vi "Filter Method Types.vi"(7 "VI Type to filter for":T2, 8 "Error in":errorcluster caption="Error in (no error)", 9 "Scope":T9, 11 "Methods":T1[](array[typedef])) -> (0 "Error out":errorcluster, 1 "All Filtered?":bool, 3 "Filtered Methods":T1[](array[typedef]))   [LabVIEW 2023, in "VIDoc Printer - Confluence.lvlib" / "VIDoc Printer - Confluence.lvclass"]
uses:
  VIDoc Printer - Confluence.lvclass
  Parsing/TypeDefs/VI Type Extended Enum.ctl
  Settings/Printer Settings/Scope Settings.ctl
  Parsing/TypeDefs/Method Spec Cluster.ctl
  <vilib>/picture/picture.llb/imagedata.ctl
  Parsing/TypeDefs/Class Dispatch Type Enum.ctl
  Parsing/TypeDefs/Controls Info Cluster.ctl
  <vilib>/Utility/miscctls.llb/LVKeyTypeDef.ctl
  <vilib>/Utility/miscctls.llb/LVPointTypeDef.ctl
  Parsing/SubVIs/Structure Reporter/Tree Cluster.ctl
  VIDoc Printer - Confluence.lvclass/VIDoc Printer - Confluence.ctl
  Parsing/VIDoc Parsing.lvlib
  Settings/Printer Settings/Printer Settings.lvclass
  Parsing/SubVIs/Structure Reporter/Structure Reporter.lvlib
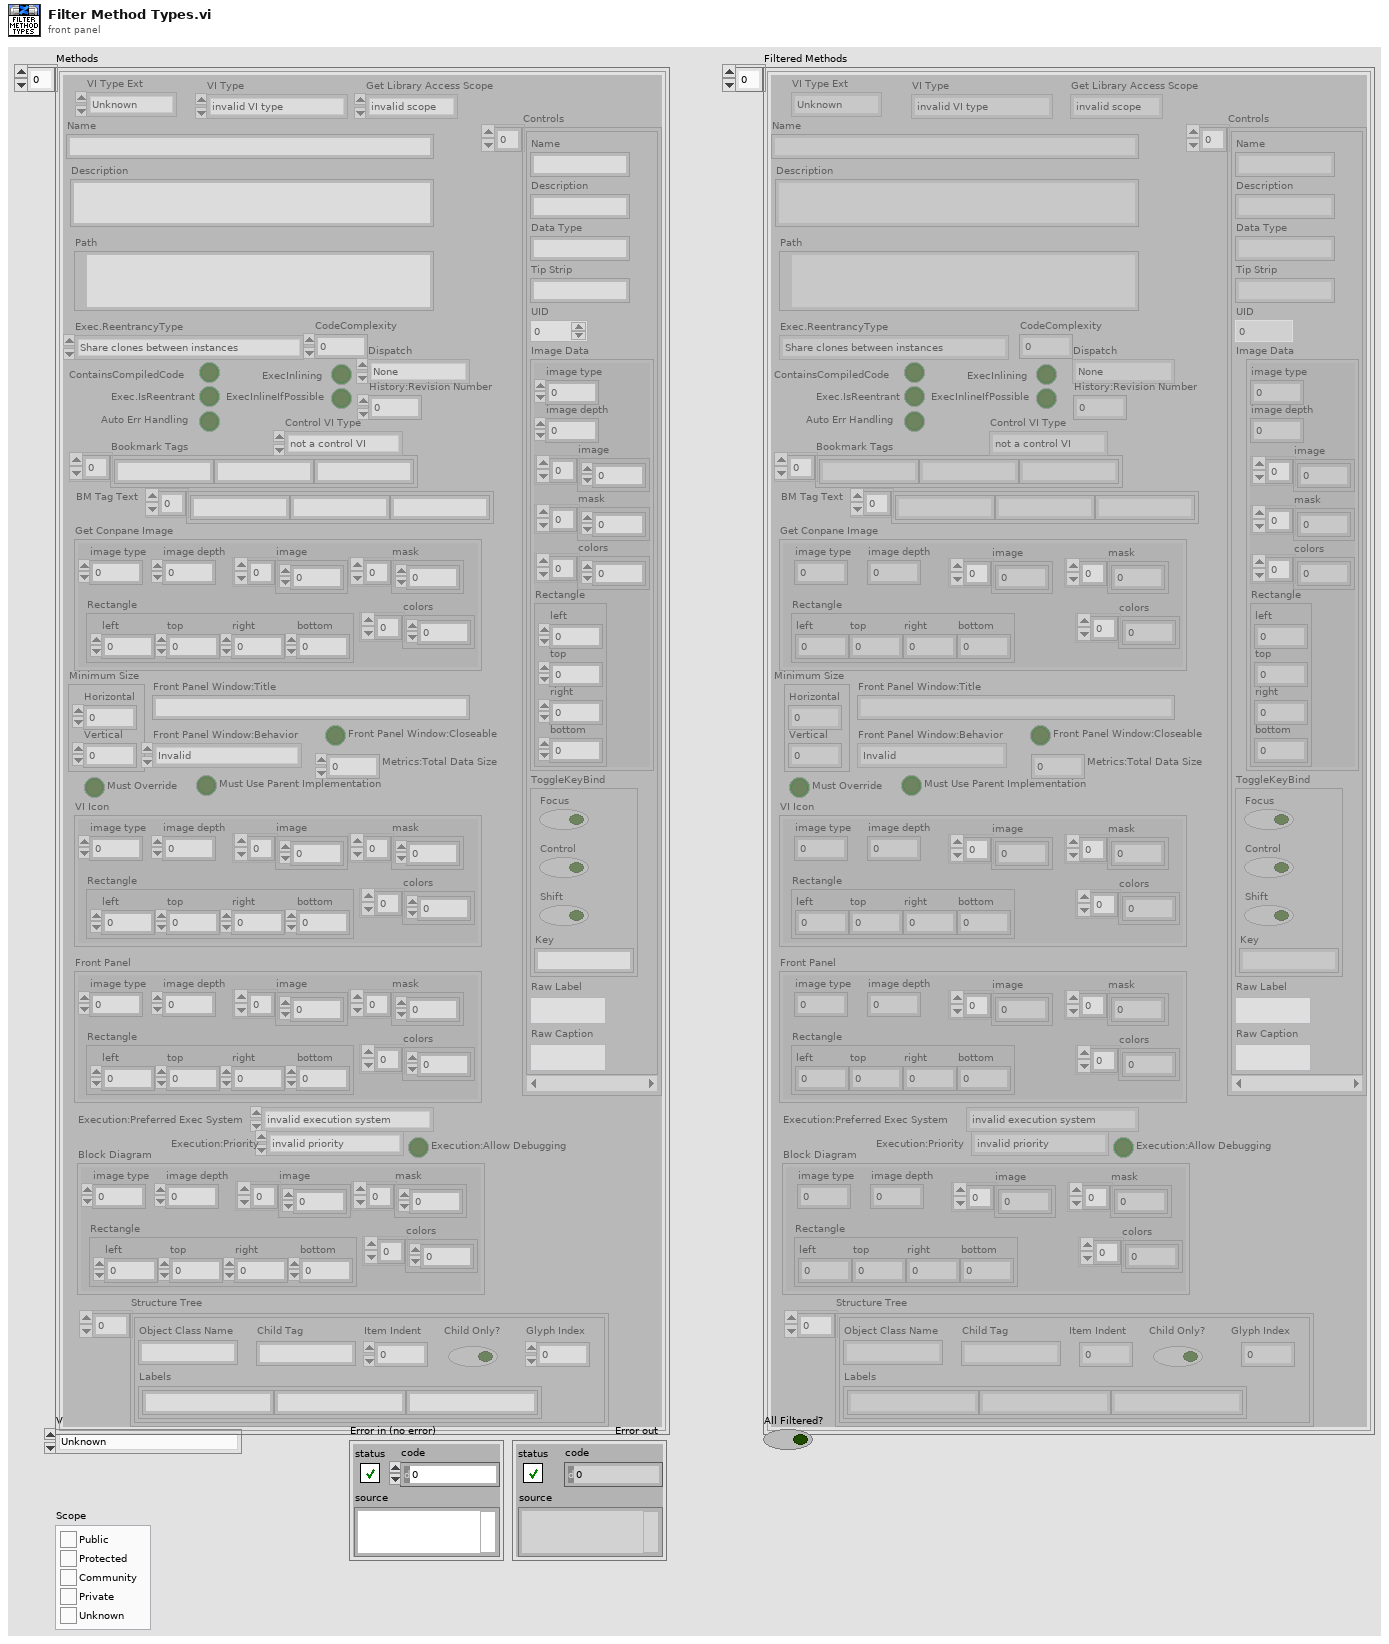
[diagram p1: front panel]
types:
  T1 = typedef "VIDoc Parsing.lvlib/Method Spec Cluster.ctl" = cluster{"VI Type Ext":T2, "Name":string, "Path":path, "Get Conpane Image":T3, "Description":string, "Get Library Access Scope":enum32{"invalid scope", "public", "private", "protected", "community"}, "Dispatch":T4, "ContainsCompiledCode":bool, "Exec.IsReentrant":bool, "Exec.ReentrancyType":enum16{"Share clones between instances", "Preallocate clone for each instance"}, "ExecInlining":bool, "ExecInlineIfPossible":bool, "Auto Err Handling":bool, "CodeComplexity":sgl, "Bookmark Tags":string[], "Control VI Type":enum32{"not a control VI", "control", "typedef", "strict typedef"}, "Controls":T5[], "VI Type":enum32{"invalid VI type", "Standard VI", "Control VI", "Global VI", "Polymorphic VI", "Configuration VI", "SubSystem", "Facade VI", "Method VI", "Statechart Diagram VI"}, "Minimum Size":T7, "Front Panel Window:Title":string, "Front Panel Window:Behavior":enum32{"Invalid", "Default", "Floating", "Floating/Auto-Hide", "Modal"}, "Front Panel Window:Closeable":bool, "Must Override":bool, "Must Use Parent Implementation":bool, "VI Icon":T3, "Front Panel":T3, "History:Revision Number":u32, "Metrics:Total Data Size":u32, "Execution:Allow Debugging":bool, "Execution:Preferred Exec System":enum32{"invalid execution system", "user interface", "standard", "instrument i/o", "data acquisition", "other 1", "other 2", "same as caller"}, "Execution:Priority":enum32{"invalid priority", "background priority", "normal priority", "above normal priority", "high priority", "time critical priority", "subroutine"}, "BM Tag Text":string[], "Block Diagram":T3, "Structure Tree":T8[]}
  T2 = typedef "VIDoc Parsing.lvlib/VI Type Extended Enum.ctl" = enum16{"Unknown", "Class Method", "Class Accessor Get", "Class Accessor Set", "Class Control", "Library Method", "Library Control", "VI", "Control"}
  T3 = typedef "imagedata.ctl" = cluster{"image type":i32, "image depth":i32, "image":u8[], "mask":u8[], "colors":u32[], "Rectangle":cluster{"left":i16, "top":i16, "right":i16, "bottom":i16}}
  T4 = typedef "VIDoc Parsing.lvlib/Class Dispatch Type Enum.ctl" = enum16{"None", "Static", "Dynamic"}
  T5 = typedef "VIDoc Parsing.lvlib/Controls Info Cluster.ctl" = cluster{"Name":string, "Description":string, "Data Type":string, "Tip Strip":string, "UID":i32, "Image Data":T3, "ToggleKeyBind":T6, "Raw Label":string, "Raw Caption":string}
  T6 = typedef "LVKeyTypeDef.ctl" = cluster{"Focus":bool, "Control":bool, "Shift":bool, "Key":string}
  T7 = typedef "LVPointTypeDef.ctl" = cluster{"Horizontal":i16, "Vertical":i16}
  T8 = typedef "VIDoc Parsing.lvlib/Structure Reporter.lvlib/Tree Cluster.ctl" = cluster{"Object Class Name":string, "Labels":string[], "Child Tag":string, "Item Indent":i32, "Child Only?":bool, "Glyph Index":i32}
  T9 = typedef "VIDoc Printer.lvlib/Printer Settings.lvclass/Scope Settings.ctl" = cluster{"Public":bool, "Protected":bool, "Community":bool, "Private":bool, "Unknown":bool}
  T10 = enum32{"invalid scope", "public", "private", "protected", "community"}
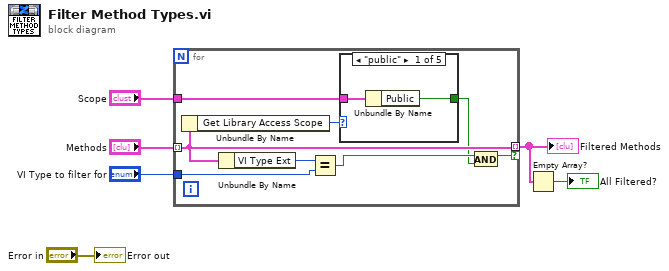
[diagram p0: block diagram]
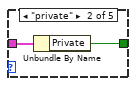
[diagram p2: hidden frame]
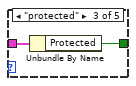
[diagram p3: hidden frame]
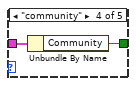
[diagram p4: hidden frame]
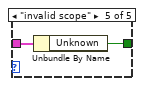
[diagram p5: hidden frame]
diagram:
  n1 = for {
    tunnel: "Methods" -> [w11] mode=indexing
    tunnel: [w11] -> w4 mode=indexing if=w9
    tunnel: "Scope" -> [w10]
    tunnel: "VI Type to filter for" -> [w7]
    n2 = Unbundle By Name(w11) -> ("Get Library Access Scope"=w12:T10)
    n3 = Unbundle By Name(w11) -> ("VI Type Ext"=w14:T2)
    n4 = Equal?(x=w14, y=w7) -> (x = y?=w13:bool)
    n5 = case shown="\"public\"" w12 {
      tunnel: w10 -> [w16 w18 w20 w22 w24]
      tunnel: [w15 w17 w19 w21 w23] -> w8
      frame "public" {
        n6 = Unbundle By Name(w16) -> ("Public"=w15:bool)
      }
      frame "private" {
        n7 = Unbundle By Name(w18) -> ("Private"=w17:bool)
      }
      frame "protected" {
        n8 = Unbundle By Name(w20) -> ("Protected"=w19:bool)
      }
      frame "community" {
        n9 = Unbundle By Name(w22) -> ("Community"=w21:bool)
      }
      frame "invalid scope" {
        n10 = Unbundle By Name(w24) -> ("Unknown"=w23:bool)
      }
    }
    n11 = And(x=w13, y=w8) -> (x .and. y?=w9:bool)
  }
  "Filtered Methods" <- w4
  n12 = Empty Array?(array=w4) -> (empty?=→"All Filtered?":bool)
  "Error out" <- "Error in"
